vi "Info.vi"(8 "error in (no error)":errorcluster, 10 "Log Text":string, 11 "Logger in":refnum<class "Logger.lvclass">) -> (0 "error out":errorcluster, 2 "Log Output":string, 3 "Logger out":refnum<class "Logger.lvclass">)   [LabVIEW 2020, in "LV Logging.lvlib" / "Logger.lvclass"]
uses:
  Logger.lvclass
  Logger.lvclass/Logger.ctl
  Type Defs/Debug Level.ctl
  LV Logging.lvlib
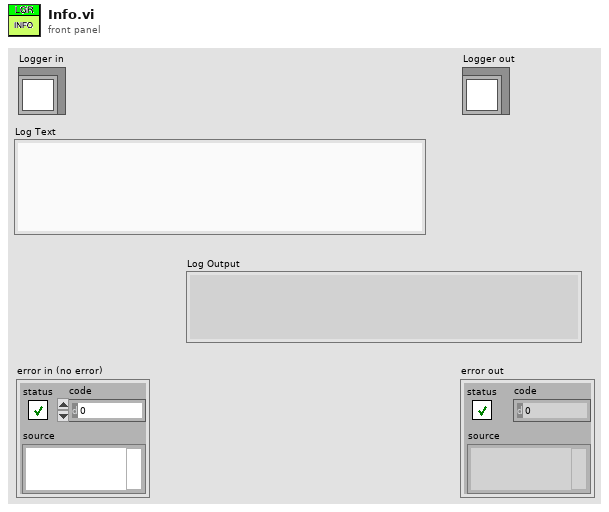
[diagram p1: front panel]
types:
  T1 = typedef "LV Logging.lvlib/Debug Level.ctl" = enum16{"DEBUG", "INFO", "WARN", "ERROR", "FATAL"}
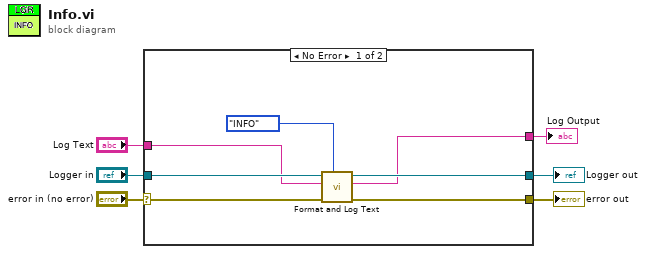
[diagram p0: block diagram]
diagram:
  n1 = case shown="No Error" "error in (no error)" {
    selector: "error in (no error)" -> [w13 w15]
    tunnel: [w12 w15] -> w5
    tunnel: [w10 w14] -> w3
    tunnel: "Logger in" -> [w11 w14]
    tunnel: "Log Text" -> [w8 _]
    tunnel: [w9 _] -> w1
    frame No Error {
      n2 = call "Format and Log Text.vi"("Debug Level"=Debug_Level."INFO" ("Debug Level out"), "error in (no error)"=w13, "Log Text"=w8, "Logger in"=w11) -> ("error out"=w12:errorcluster, "Log Output"=w9:string, "Logger out"=w10:refnum<class "Logger.lvclass">)  [unwired: 5 in]
    }
    frame Error {
    }
  }
  "error out" <- w5
  "Logger out" <- w3
  "Log Output" <- w1
